vi "APS get nv ram.vi"(6 "Data":i32, 7 "Offset":i32, 8 "error in (no error)":errorcluster caption="错误输入（无错误）", 9 "DataWidth":i32, 10 "RamNo":i32, 11 "Board_ID":i32) -> (0 "error out":errorcluster caption="错误输出", 3 "function return":i32, 4 "Data out":i32)   [LabVIEW 2011, in "APS168.lvlib"]
doc: "I32 FNTYPE APS_get_nv_ram( I32 Board_ID, I32 RamNo, I32 DataWidth, I32 Offset, I32 *Data );"
uses:
  APS168.lvlib
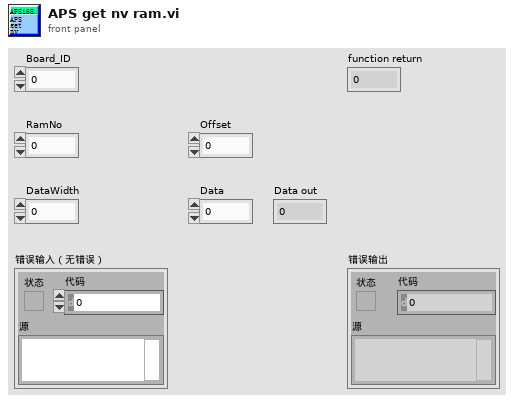
[diagram p1: front panel]
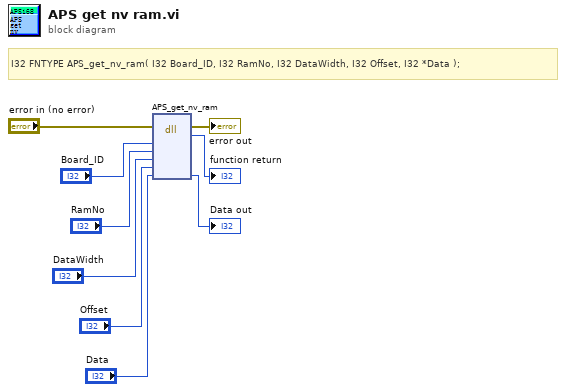
[diagram p0: block diagram]
diagram:
  # "I32 FNTYPE APS_get_nv_ram( I32 Board_ID, I32 RamNo, I32 DataWidth, I32 Offset, I32 *Data );"
  n1 = dll-call lib="PTH1Labs E软件ADLINK 204CAPS_1_7_1_LIB line 连续运动204APS168.*" fn="APS_get_nv_ram"(error in="error in (no error)", "Board_ID"="Board_ID", "RamNo"="RamNo", "DataWidth"="DataWidth", "Offset"="Offset", "Data"="Data") -> (error out=→"error out":errorcluster, →"function return":i32, "Data"=→"Data out":i32)  [unwired: 6 in, 1 out]
